vi "Stop delay.vi"(8 "error in (no error)":errorcluster, 10 "Period (ms)":dbl, 11 "Delay (s)":dbl) -> (0 "error out":errorcluster, 2 "Remaining delay":dbl, 3 "Stop?":bool)   [LabVIEW 2017]
panel:
  # "VI Description: Outputs a boolean \"stop\" to instruct the motors to stop for a period of time specified by\nthe 'Delay' control. This VI is necessary to allow the rest of the loop to continue running as normal, instead\nof forcing the whole program to stop while the motors stop.\nThe VI uses a Functional Global Variable to store the values of the previous delay, so that the delay is slowly\nreduced until it hits 0 as the main loop continues to run.\nThis VI also prevents timing errors that would occur in PID loops if a standard \"wait\" delay was used in the\ntop level."
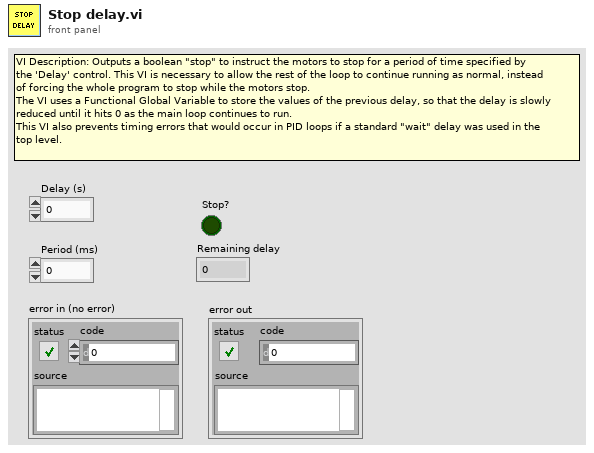
[diagram p1: front panel]
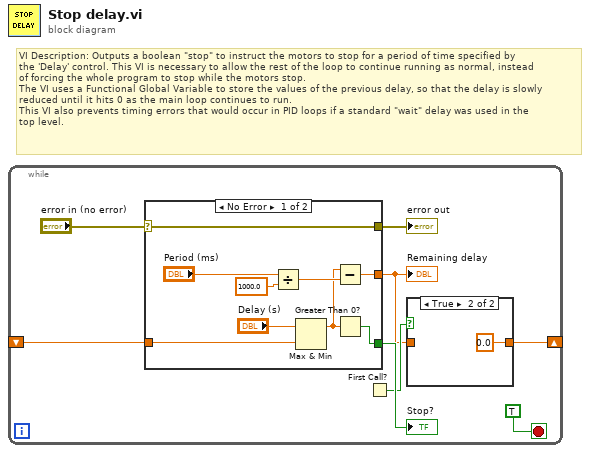
[diagram p0: block diagram]
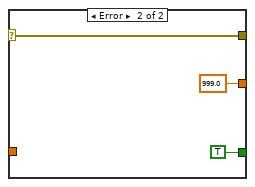
[diagram p3: hidden frame]
diagram:
  # "VI Description: Outputs a boolean \"stop\" to instruct the motors to stop for a period of time specified by\nthe 'Delay' control. This VI is necessary to allow the rest of the loop to continue running as normal, instead\nof forcing the whole program to stop while the motors stop.\nThe VI uses a Functional Global Variable to store the values of the previous delay, so that the delay is slowly\nreduced until it hits 0 as the main loop continues to run.\nThis VI also prevents timing errors that would occur in PID loops if a standard \"wait\" delay was used in the\ntop level."
  n1 = while {
    shift-right: [w1] -> _
    shift-left: _ -> [w6]
    stop <- TRUE stop-if-true
    n2 = case shown="No Error" "error in (no error)" {
      selector: "error in (no error)" -> [w11 w20]
      tunnel: [w18 TRUE] -> w7
      tunnel: [w13 999.0] -> w2
      tunnel: w6 -> [w12 _]
      tunnel: [w11 w20] -> w4
      frame No Error {
        n3 = Divide(x="Period (ms)", y=1000.0) -> (x/y=w15:dbl)
        n4 = Max & Min(x="Delay (s)", y=w12) -> (max(x,y)=w14:dbl)  [unwired: 1 out]
        n5 = Subtract(x=w14, y=w15) -> (x-y=w13:dbl)
        n6 = Greater Than 0?(x=w14) -> (x > 0?=w18:bool)
      }
      frame Error {
      }
    }
    "Stop?" <- w7
    "Remaining delay" <- w2
    "error out" <- w4
    n7 = First Call?() -> (First Call?: T/F=w3:bool)
    n8 = case shown="True" w3 {
      tunnel: w2 -> [w9 _]
      tunnel: [w9 0.0] -> w1
      frame False {
      }
      frame True {
      }
    }
  }
